vi "Ping Actor.vi"(8 "error in (no error)":errorcluster, 9 "Timeout if waiting(-1ms)":i32=-1, 10 "Actor in":refnum<class "Actor.lvclass">, 11 "Target Enqueuer":refnum<class "Message Enqueuer.lvclass">) -> (0 "error out":errorcluster, 3 "Success?":bool)   [LabVIEW 2020, in "Publisher.lvlib" / "Ping Msg.lvclass"]
doc: "Send a Ping Msg on an enqueuer and wait for the response."
uses:
  Ping Msg.lvclass
  PPL/HDH.Actor Framework.Core.Actor.lvlibp/1abvi3w/vi.lib/ActorFramework/Message Enqueuer/Message Enqueuer.lvclass
  PPL/HDH.Actor Framework.Core.Actor.lvlibp/1abvi3w/vi.lib/ActorFramework/Actor/Actor.lvclass
  C:/Current projects/WS/Framework/Framework/Actors/Publisher/Messages/Response Msg/Response Msg.lvclass
  Response Msg/Response Core/Controls/Ctl_SendFunction.ctl
  PPL/HDH.Actor Framework.Core.Actor.lvlibp/1abvi3w/vi.lib/ActorFramework/Message Enqueuer/Message Priority.ctl
  Publisher Messages/Bypass Msg/Bypass Msg.lvclass/Bypass Msg.ctl
  Publisher Messages/Bypass Msg/Bypass Msg.lvclass
  C:/Current projects/WS/Framework/Framework/Actors/Publisher/Publisher Messages/Sender Msg/Sender Msg.lvclass
  Response Msg/Response Msg.lvclass
  Publisher.lvlib
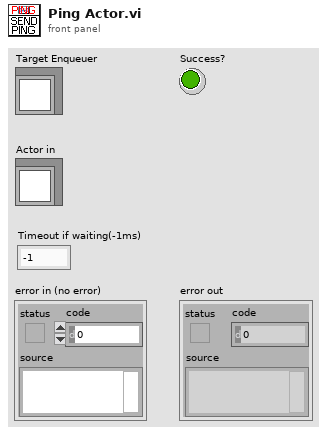
[diagram p1: front panel]
types:
  T1 = typedef "HDH.Actor Framework.Core.Actor.lvlibp/Message Enqueuer.lvclass/Message Priority.ctl" = enum16{"Low", "Normal", "High"}
  T2 = typedef "Publisher.lvlib/Ctl_SendFunction.ctl" = enum16{"Send and Forget", "Request Reply", "Await Reply"}
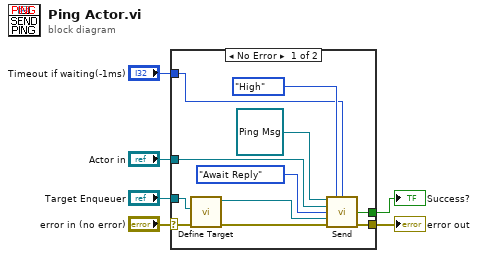
[diagram p0: block diagram]
diagram:
  n1 = case shown="No Error" "error in (no error)" {
    selector: "error in (no error)" -> [w16 w18]
    tunnel: [w8 w18] -> w5
    tunnel: "Target Enqueuer" -> [w17 _]
    tunnel: "Timeout if waiting(-1ms)" -> [w11 _]
    tunnel: [w9 _] -> w2
    tunnel: "Actor in" -> [w7 _]
    frame No Error {
      n2 = call "Define Target.vi"("error in (no error)"=w16, "Target Enqueuer"=w17) -> ("error out"=w10:errorcluster, "Targetted Msg out"=w15:refnum<class "Bypass Msg.lvclass">)  [unwired: 8 in]
      n3 = call "Send.vi"("Response Msg in"=refnum<class "Ping Msg.lvclass"> refnum ("Publisher.lvlib:Ping Msg.lvclass"), "Message Priority (Normal)"=Message_Priority."High", "Timeout if waiting(-1ms)"=w11, "Actor in"=w7, "Send Function"=Ctl_SendFunction."Await Reply", "Sender (publish)"=w15, "error in (no error)"=w10) -> ("Success?"=w9:bool, "error out"=w8:errorcluster)  [unwired: 4 in, 3 out]
    }
    frame Error {
    }
  }
  "error out" <- w5
  "Success?" <- w2
